vi "I2C_Busses.vi"(6 "error in":errorcluster) -> (0 "error out":errorcluster, 4 "I2C Busses":i32[](array[numeric]))   [LabVIEW 2014]
doc: "Scans for available I2C buses"
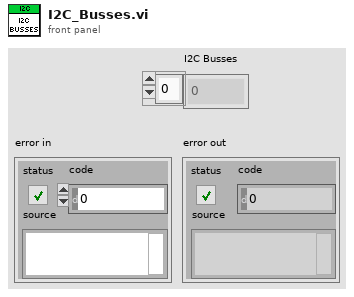
[diagram p1: front panel]
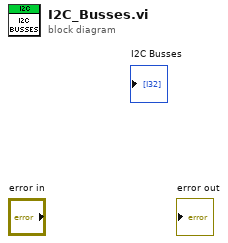
[diagram p0: block diagram]
diagram:
